vi "create communicator task.vi"(8 "error in":errorcluster, 10 "queue size (1,10000)":i32, 11 "communicator":refnum<class "communicator.lvclass">) -> (0 "error out":errorcluster, 3 "communicator task out":refnum<class "communicator task.lvclass">)   [LabVIEW 2015, in "communicator task.lvclass"]
uses:
  communicator task.lvclass
  communicator/communicator.lvclass
  communicator task.lvclass/communicator task.ctl
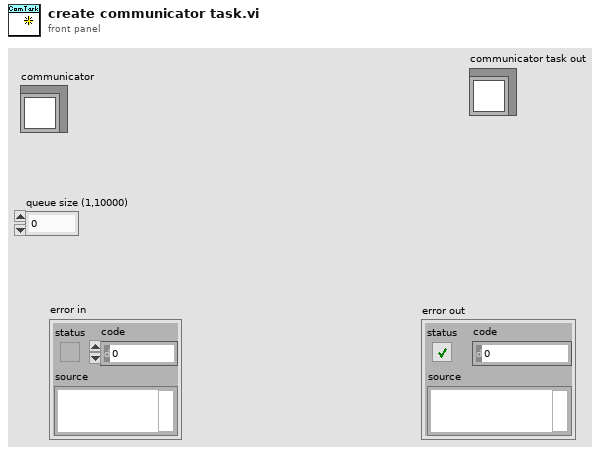
[diagram p1: front panel]
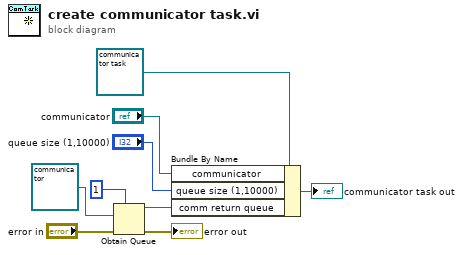
[diagram p0: block diagram]
diagram:
  n1 = Obtain Queue(max queue size (-1, unlimited)=1, element data type=refnum<class "communicator.lvclass"> refnum ("communicator in"), error in (no error)="error in") -> (queue out=w1:refnum<queue>, error out=→"error out":errorcluster)  [unwired: 2 in, 1 out]
  n2 = Bundle By Name(cluster=refnum<class "communicator task.lvclass"> refnum ("communicator task in"), "communicator"="communicator", "queue size (1,10000)"="queue size (1,10000)", "comm return queue"=w1) -> (→"communicator task out":refnum<class "communicator task.lvclass">)
